vi "Write Control Height.vi"(8 "error in":errorcluster, 10 "Height":u32, 11 "Control in":refnum<vi>) -> (0 "error out":errorcluster, 3 "Control":refnum<vi>)   [LabVIEW 2020, in "VolatusGUIEditorCore.lvlib"]
uses:
  VolatusGUIEditorCore.lvlib
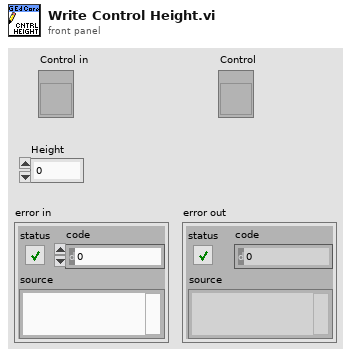
[diagram p1: front panel]
types:
  T1 = typedef "LVBoundsTypeDef.ctl" = cluster{"Width":u32, "Height":u32}
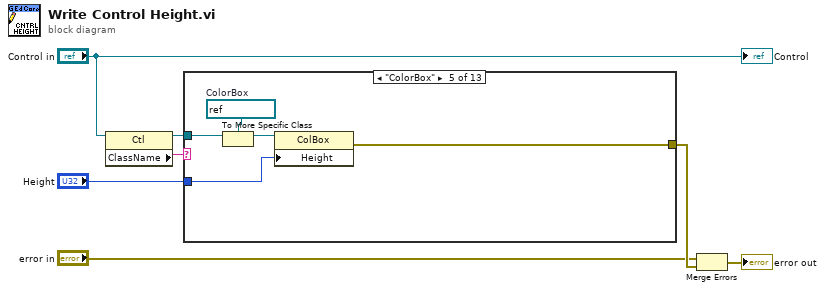
[diagram p0: block diagram]
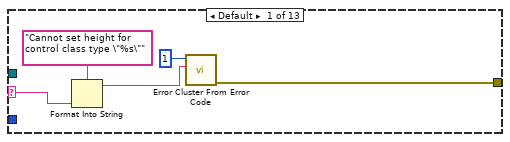
[diagram p2: hidden frame]
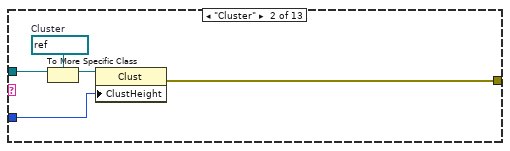
[diagram p3: hidden frame]
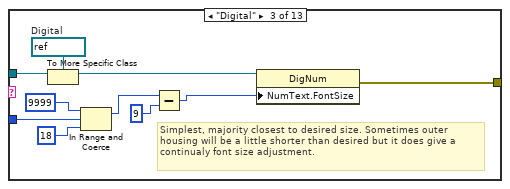
[diagram p4: hidden frame]
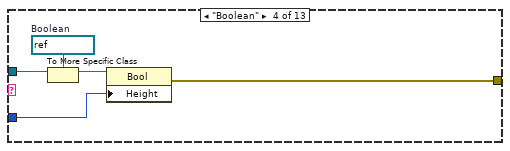
[diagram p5: hidden frame]
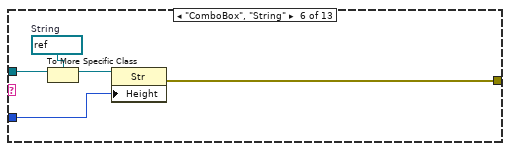
[diagram p6: hidden frame]
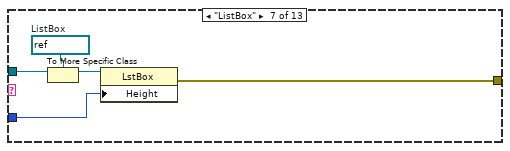
[diagram p7: hidden frame]
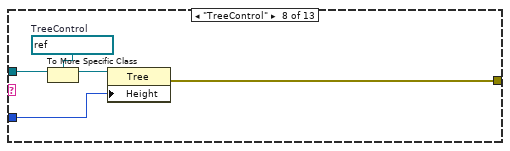
[diagram p8: hidden frame]
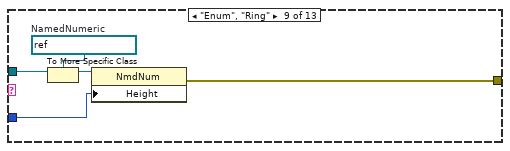
[diagram p9: hidden frame]
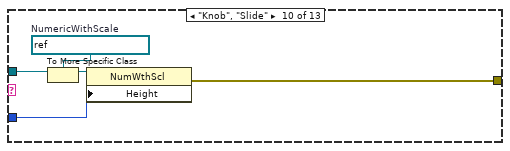
[diagram p10: hidden frame]
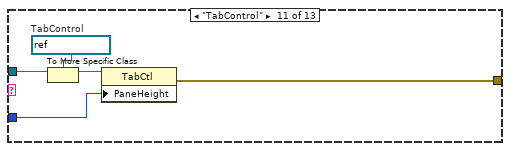
[diagram p11: hidden frame]
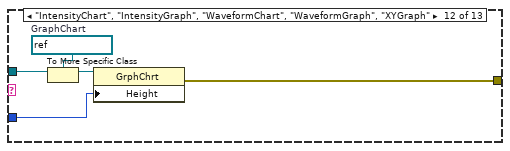
[diagram p12: hidden frame]
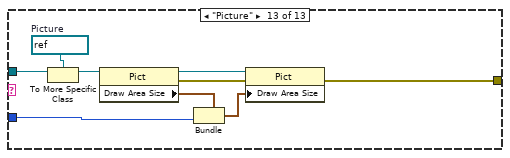
[diagram p13: hidden frame]
diagram:
  n1 = property class="Ctl"(reference="Control in") -> (reference out=w6:refnum<vi>, "ClassName"=w7:string)  [unwired: 1 in, 1 out]
  n2 = case shown="\"ColorBox\"" w7 {
    selector: w7 -> [w9 _ _ _ _ _ _ _ _ _ _ _ _]
    tunnel: w6 -> [_ w17 w27 w32 w37 w42 w47 w52 w57 w62 w67 w72 w81]
    tunnel: "Height" -> [_ w14 w21 w29 w34 w39 w44 w49 w54 w59 w64 w69 w73]
    tunnel: [w12 w13 w24 w28 w33 w38 w43 w48 w53 w58 w63 w68 w74] -> w3
    frame Default {
      n3 = Format Into String(format string="Cannot set height for control class type \"%s\"", w9) -> (resulting string=w8:string)  [unwired: 2 in, 1 out]
      n4 = call <vilib>:"Error Cluster From Error Code.vi"("error message (\"\")"=w8, "error code (0)"=1) -> ("error out"=w12:errorcluster)  [unwired: 7 in]
    }
    frame "Cluster" {
      w16 = refnum<vi> refnum  # Cluster
      n5 = To More Specific Class(target class=w16, reference=w17) -> (specific class reference=w15:refnum<vi>)  [unwired: 1 in, 1 out]
      n6 = property class="Clust"(reference=w15, "ClustHeight"=w14) -> (error out=w13:errorcluster)  [unwired: 1 in, 1 out]
    }
    frame "Digital" {
      w26 = refnum<vi> refnum  # Digital
      # "Simplest, majority closest to desired size. Sometimes outer housing will be a little shorter than desired but it does give a continualy font size adjustment."
      n7 = To More Specific Class(target class=w26, reference=w27) -> (specific class reference=w25:refnum<vi>)  [unwired: 1 in, 1 out]
      n8 = In Range and Coerce(upper limit=u32 9999, x=w21, lower limit=u32 18) -> (coerced(x)=w19:u32)  [unwired: 1 out]
      n9 = Subtract(x=w19, y=u32 9) -> (x-y=w23:u32)
      n10 = property class="DigNum"(reference=w25, "NumText.FontSize"=w23) -> (error out=w24:errorcluster)  [unwired: 1 in, 1 out]
    }
    frame "Boolean" {
      w31 = refnum<vi> refnum  # Boolean
      n11 = To More Specific Class(target class=w31, reference=w32) -> (specific class reference=w30:refnum<vi>)  [unwired: 1 in, 1 out]
      n12 = property class="Bool"(reference=w30, "Height"=w29) -> (error out=w28:errorcluster)  [unwired: 1 in, 1 out]
    }
    frame "ColorBox" {
      w36 = refnum<vi> refnum  # ColorBox
      n13 = To More Specific Class(target class=w36, reference=w37) -> (specific class reference=w35:refnum<vi>)  [unwired: 1 in, 1 out]
      n14 = property class="ColBox"(reference=w35, "Height"=w34) -> (error out=w33:errorcluster)  [unwired: 1 in, 1 out]
    }
    frame "ComboBox", "String" {
      w41 = refnum<vi> refnum  # String
      n15 = To More Specific Class(target class=w41, reference=w42) -> (specific class reference=w40:refnum<vi>)  [unwired: 1 in, 1 out]
      n16 = property class="Str"(reference=w40, "Height"=w39) -> (error out=w38:errorcluster)  [unwired: 1 in, 1 out]
    }
    frame "ListBox" {
      w46 = refnum<vi> refnum  # ListBox
      n17 = To More Specific Class(target class=w46, reference=w47) -> (specific class reference=w45:refnum<vi>)  [unwired: 1 in, 1 out]
      n18 = property class="LstBox"(reference=w45, "Height"=w44) -> (error out=w43:errorcluster)  [unwired: 1 in, 1 out]
    }
    frame "TreeControl" {
      w51 = refnum<vi> refnum  # TreeControl
      n19 = To More Specific Class(target class=w51, reference=w52) -> (specific class reference=w50:refnum<vi>)  [unwired: 1 in, 1 out]
      n20 = property class="Tree"(reference=w50, "Height"=w49) -> (error out=w48:errorcluster)  [unwired: 1 in, 1 out]
    }
    frame "Enum", "Ring" {
      w56 = refnum<vi> refnum  # NamedNumeric
      n21 = To More Specific Class(target class=w56, reference=w57) -> (specific class reference=w55:refnum<vi>)  [unwired: 1 in, 1 out]
      n22 = property class="NmdNum"(reference=w55, "Height"=w54) -> (error out=w53:errorcluster)  [unwired: 1 in, 1 out]
    }
    frame "Knob", "Slide" {
      w61 = refnum<vi> refnum  # NumericWithScale
      n23 = To More Specific Class(target class=w61, reference=w62) -> (specific class reference=w60:refnum<vi>)  [unwired: 1 in, 1 out]
      n24 = property class="NumWthScl"(reference=w60, "Height"=w59) -> (error out=w58:errorcluster)  [unwired: 1 in, 1 out]
    }
    frame "TabControl" {
      w66 = refnum<vi> refnum  # TabControl
      n25 = To More Specific Class(target class=w66, reference=w67) -> (specific class reference=w65:refnum<vi>)  [unwired: 1 in, 1 out]
      n26 = property class="TabCtl"(reference=w65, "PaneHeight"=w64) -> (error out=w63:errorcluster)  [unwired: 1 in, 1 out]
    }
    frame "IntensityChart", "IntensityGraph", "WaveformChart", "WaveformGraph", "XYGraph" {
      w71 = refnum<vi> refnum  # GraphChart
      n27 = To More Specific Class(target class=w71, reference=w72) -> (specific class reference=w70:refnum<vi>)  [unwired: 1 in, 1 out]
      n28 = property class="GrphChrt"(reference=w70, "Height"=w69) -> (error out=w68:errorcluster)  [unwired: 1 in, 1 out]
    }
    frame "Picture" {
      w80 = refnum<vi> refnum  # Picture
      n29 = To More Specific Class(target class=w80, reference=w81) -> (specific class reference=w79:refnum<vi>)  [unwired: 1 in, 1 out]
      n30 = property class="Pict"(reference=w79) -> (reference out=w77:refnum<vi>, error out=w75:errorcluster, "Draw Area Size"=w78:T1)  [unwired: 1 in]
      n31 = Bundle(cluster=w78, "Height"=w73) -> (w76:T1)  [unwired: 1 in]
      n32 = property class="Pict"(reference=w77, error in=w75, "Draw Area Size"=w76) -> (error out=w74:errorcluster)  [unwired: 1 out]
    }
  }
  n33 = Merge Errors("error in", w3) -> (→"error out":errorcluster)
  "Control" <- "Control in"
